vi "collectFrame.vi"(7 "Reset":bool, 8 "error in (no error)":errorcluster, 10 "byte":u8, 11 "RTU in":refnum<class "RTU.lvclass">) -> (0 "error out":errorcluster, 1 "Data":i16[](array[numeric]), 2 "Finished":bool, 3 "RTU out":refnum<class "RTU.lvclass">, 5 "OK?":bool)   [LabVIEW 2015, in "ModBUS.lvlib" / "RTU.lvclass"]
uses:
  RTU.lvclass
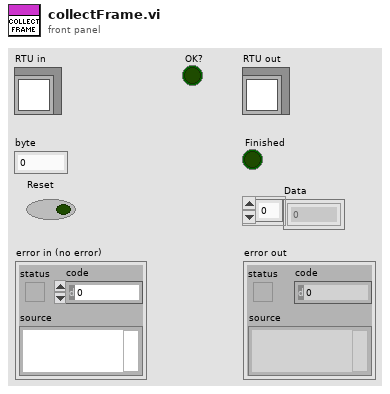
[diagram p1: front panel]
types:
  T1 = cluster{"SlaveAddress":u8, "FunctionCode":u8, "DataAddress":u16, "byteCount":u8, "Data":i16[], "CRC":u16, "wordsToRead":u8, "DataItem":i16}
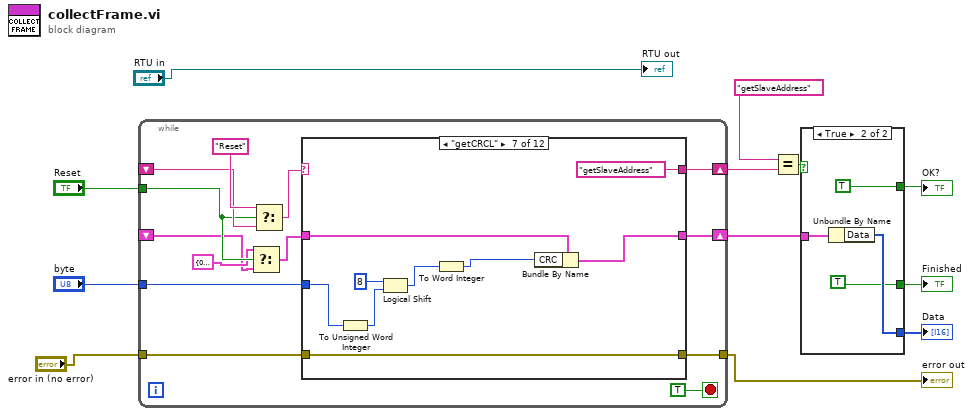
[diagram p0: block diagram]
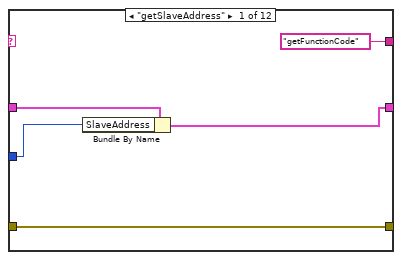
[diagram p3: hidden frame]
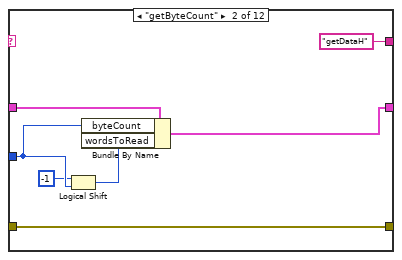
[diagram p4: hidden frame]
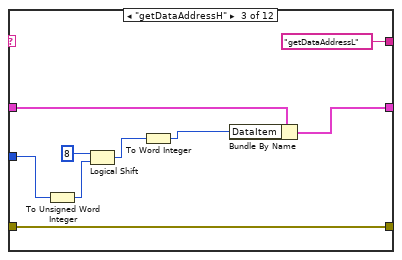
[diagram p5: hidden frame]
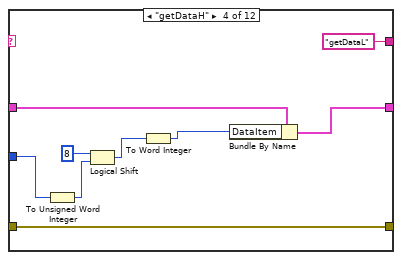
[diagram p6: hidden frame]
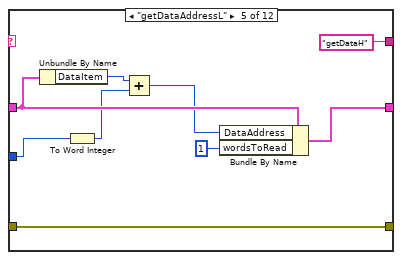
[diagram p7: hidden frame]
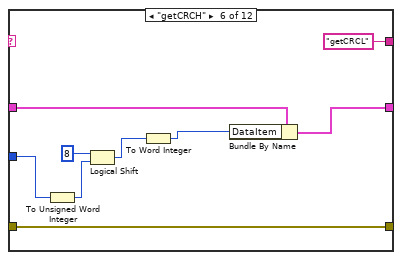
[diagram p8: hidden frame]
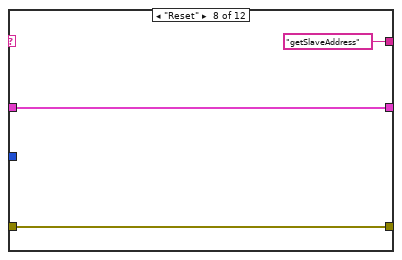
[diagram p9: hidden frame]
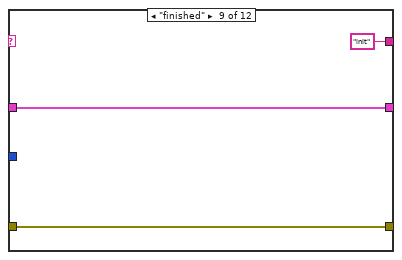
[diagram p10: hidden frame]
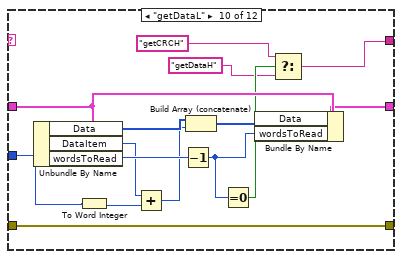
[diagram p11: hidden frame]
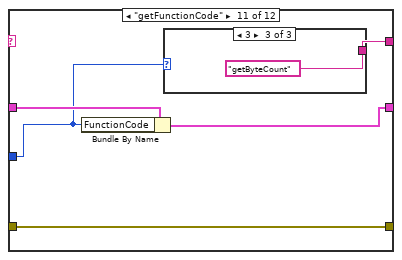
[diagram p12: hidden frame]
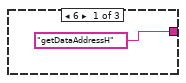
[diagram p13: hidden frame]
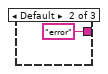
[diagram p14: hidden frame]
diagram:
  n1 = while {
    tunnel: "error in (no error)" -> [w25]
    tunnel: [w24] -> w10
    shift-right: [w23] -> w7
    shift-left: _ -> [w21]
    tunnel: "Reset" -> [w16]
    tunnel: "byte" -> [w19]
    shift-right: [w18] -> w4
    shift-left: _ -> [w14]
    stop <- TRUE stop-if-true
    n2 = Select(t=T1 {"SlaveAddress"=0, "FunctionCode"=0, "DataAddress"=0, "byteCount"=0, "Data"=[], "CRC"=0, "wordsToRead"=0, "DataItem"=0} ("output cluster"), s=w16, f=w14) -> (s? t:f=w13:T1)
    n3 = Select(t="Reset", s=w16, f=w21) -> (s? t:f=w20:string)
    n4 = case shown="\"getCRCL\"" w20 {
      selector: w20 -> [_ _ _ _ _ _ _ _ _ _ _ w113]
      tunnel: w25 -> [w26 w31 w42 w51 w62 w69 w78 w83 w87 w99 w104 w114]
      tunnel: [w26 w31 w42 w51 w62 w69 w78 w83 w87 w99 w104 w114] -> w24
      tunnel: ["getFunctionCode" ("t") "getDataH" ("t") "getDataAddressL" ("t") "getDataL" ("t") "getDataH" ("t") "getCRCL" ("t") "getSlaveAddress" ("t") "getSlaveAddress" ("t") "init" ("t") w89 w106 w113] -> w23
      tunnel: w19 -> [w28 w34 w41 w50 w61 w68 w77 _ _ w97 w105 _]
      tunnel: [w29 w36 w44 w53 w63 w71 w80 w84 w86 w102 w107 w112] -> w18
      tunnel: w13 -> [w30 w37 w45 w54 w59 w72 w81 w84 w86 w103 w108 w112]
      frame "getSlaveAddress" {
        n5 = Bundle By Name(cluster=w30, "SlaveAddress"=w28) -> (w29:T1)
      }
      frame "getByteCount" {
        n6 = Logical Shift(y=i16 -1, x=w34) -> (x << y=w32:u8)
        n7 = Bundle By Name(cluster=w37, "byteCount"=w34, "wordsToRead"=w32) -> (w36:T1)
      }
      frame "getDataAddressH" {
        n8 = To Unsigned Word Integer(number=w41) -> (unsigned 16bit integer=w40:u16)
        n9 = Logical Shift(y=i16 8, x=w40) -> (x << y=w39:u16)
        n10 = To Word Integer(number=w39) -> (16bit integer=w38:i16)
        n11 = Bundle By Name(cluster=w45, "DataItem"=w38) -> (w44:T1)
      }
      frame "getDataH" {
        n12 = To Unsigned Word Integer(number=w50) -> (unsigned 16bit integer=w49:u16)
        n13 = Logical Shift(y=i16 8, x=w49) -> (x << y=w48:u16)
        n14 = To Word Integer(number=w48) -> (16bit integer=w47:i16)
        n15 = Bundle By Name(cluster=w54, "DataItem"=w47) -> (w53:T1)
      }
      frame "getDataAddressL" {
        n16 = Unbundle By Name(w59) -> ("DataItem"=w58:i16)
        n17 = To Word Integer(number=w61) -> (16bit integer=w57:i16)
        n18 = Add(x=w58, y=w57) -> (x+y=w56:i16)
        n19 = Bundle By Name(cluster=w59, "DataAddress"=w56, "wordsToRead"=u8 1) -> (w63:T1)
      }
      frame "getCRCH" {
        n20 = To Unsigned Word Integer(number=w68) -> (unsigned 16bit integer=w67:u16)
        n21 = Logical Shift(y=i16 8, x=w67) -> (x << y=w66:u16)
        n22 = To Word Integer(number=w66) -> (16bit integer=w65:i16)
        n23 = Bundle By Name(cluster=w72, "DataItem"=w65) -> (w71:T1)
      }
      frame "getCRCL" {
        n24 = To Unsigned Word Integer(number=w77) -> (unsigned 16bit integer=w76:u16)
        n25 = Logical Shift(y=i16 8, x=w76) -> (x << y=w75:u16)
        n26 = To Word Integer(number=w75) -> (16bit integer=w74:i16)
        n27 = Bundle By Name(cluster=w81, "CRC"=w74) -> (w80:T1)
      }
      frame "Reset" {
      }
      frame "finished" {
      }
      frame "getDataL" {
        n28 = Unbundle By Name(w103) -> ("Data"=w101:i16[], "DataItem"=w95:i16, "wordsToRead"=w98:u8)
        n29 = To Word Integer(number=w97) -> (16bit integer=w96:i16)
        n30 = Add(x=w95, y=w96) -> (x+y=w94:i16)
        n31 = Decrement(x=w98) -> (x-1=w93:u8)
        n32 = Build Array (concatenate)(w101, w94) -> (w100:i16[])
        n33 = Equal To 0?(x=w93) -> (x = 0?=w92:bool)
        n34 = Bundle By Name(cluster=w103, "Data"=w100, "wordsToRead"=w93) -> (w102:T1)
        n35 = Select(t="getCRCH", s=w92, f="getDataH" ("t")) -> (s? t:f=w89:string)
      }
      frame "getFunctionCode" {
        n36 = Bundle By Name(cluster=w108, "FunctionCode"=w105) -> (w107:T1)
        n37 = case shown="3" w105 {
          tunnel: ["getDataAddressH" ("t") "error" ("t") "getByteCount" ("t")] -> w106
          frame 6 {
          }
          frame Default {
          }
          frame 3 {
          }
        }
      }
      frame "exit", Default {
      }
    }
  }
  "error out" <- w10
  n38 = Equal?(x="getSlaveAddress" ("t"), y=w7) -> (x = y?=w5:bool)
  n39 = case shown="True" w5 {
    tunnel: w4 -> [_ w118]
    tunnel: [_ w117] -> w3
    tunnel: [_ TRUE] -> w2
    tunnel: [_ TRUE] -> w1
    frame False {
    }
    frame True {
      n40 = Unbundle By Name(w118) -> ("Data"=w117:i16[])
    }
  }
  "Data" <- w3
  "Finished" <- w2
  "OK?" <- w1
  "RTU out" <- "RTU in"
